vi "Measure_VCOM.vi"(8 "error in (no error)":errorcluster) -> (0 "error out":errorcluster, 3 "Voltage":dbl=-0.0818253011 format="%0.8f")   [LabVIEW 2015]
doc: "This VI measure power supplies from the Modis Charger Main Board with Keithley DMM."
panel:
  in  "Sample Count":i32=1
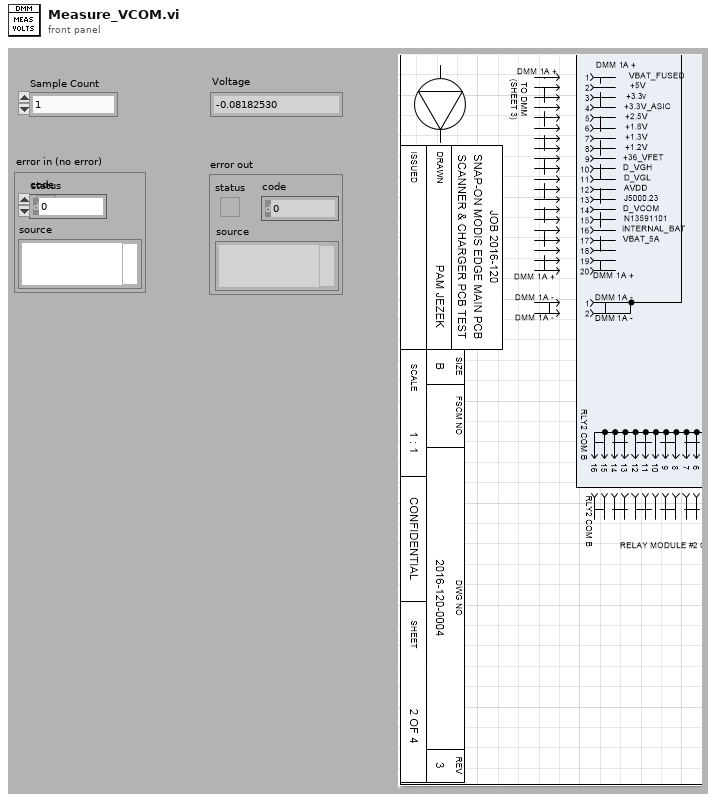
[diagram p1: front panel]
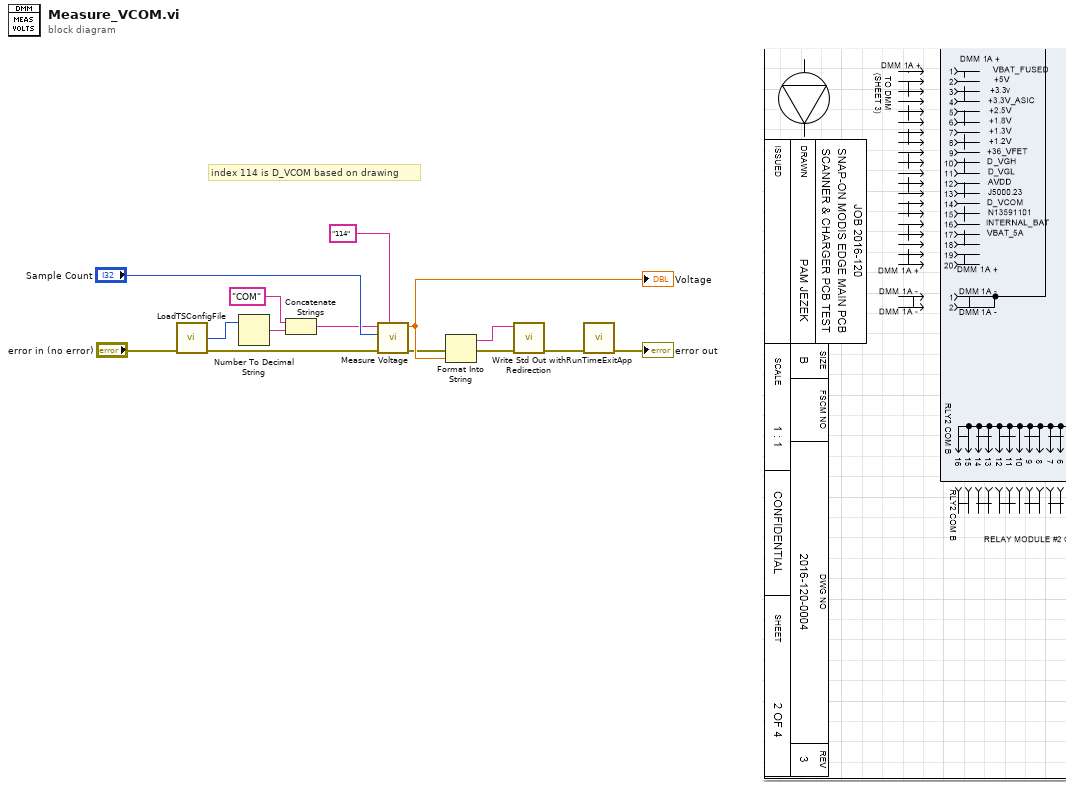
[diagram p0: block diagram]
diagram:
  # "index 114 is D_VCOM based on drawing"
  n1 = call "LoadTSConfigFile.vi"("error in (no error)"="error in (no error)") -> ("DMM_COMPort"=w11:i32, "error out"=w10:errorcluster)  [unwired: 4 in, 9 out]
  n2 = Number To Decimal String(number=w11) -> (decimal integer string=w12:string)  [unwired: 1 in]
  n3 = Concatenate Strings("COM" ("string"), w12) -> (w8:string)
  n4 = call "Measure Voltage.vi"("Channel List (101:110)"="114", "error in (no error)"=w10, "Sample Count"="Sample Count", "VISA resource name"=w8) -> ("error out"=w4:errorcluster, "Voltage"=w5:dbl)  [unwired: 5 in, 1 out]
  "Voltage" <- w5
  n5 = Format Into String(error in=w4, w5) -> (resulting string=w2:string, error out=w3:errorcluster)  [unwired: 2 in]
  n6 = call "Write Std Out with Redirection.vi"("error in (no error)"=w3, "string"=w2) -> ("error out"=w6:errorcluster)  [unwired: 9 in]
  n7 = call "RunTimeExitApp.vi"("error in (no error)"=w6) -> ("error out"=→"error out":errorcluster)  [unwired: 10 in]
